vi "tag select data type change.vi"(8 "error in":errorcluster, 9 "Dt Value":i32, 10 "tag select":string, 11 "object ref in":T1) -> (0 "error out":errorcluster, 3 "object ref out":T1)   [LabVIEW 2013, in "tag select module editor node.lvclass"]
uses:
  tag select module editor node.lvclass
  object ref.ctl
  <vilib>/NI/Tag Bus Data Framework/Configuration Editor/Classes/Engine Parent/Engine Parent Editor Node.lvclass
  module/configuration/tag select module configuration.lvclass
  <vilib>/NI/Configuration Framework/serializable configuration/NISE_CEF_serializable configuration.lvclass/NISE_CEF_serializable configuration.ctl
  <vilib>/Utility/LVClass/Get LV Class Name.vi
  <vilib>/NI/Configuration Framework/error generator/NISE_error generator.vi
  <vilib>/NI/Module Execution Interface/Engine Configuration/engine configuration.lvclass
  <vilib>/NI/Configuration Framework/serializable configuration/NISE_CEF_serializable configuration.lvclass
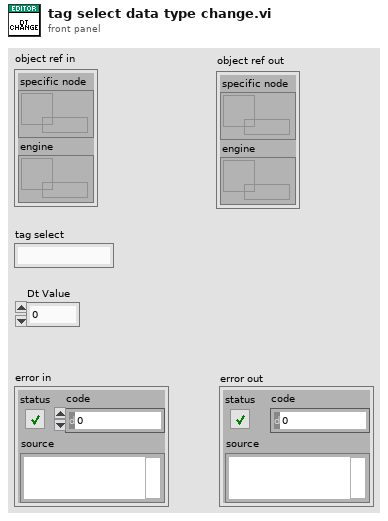
[diagram p1: front panel]
types:
  T1 = typedef "tag select module editor node.lvclass/object ref.ctl" = cluster{"specific node":refnum<data-value>, "engine":refnum<data-value>}
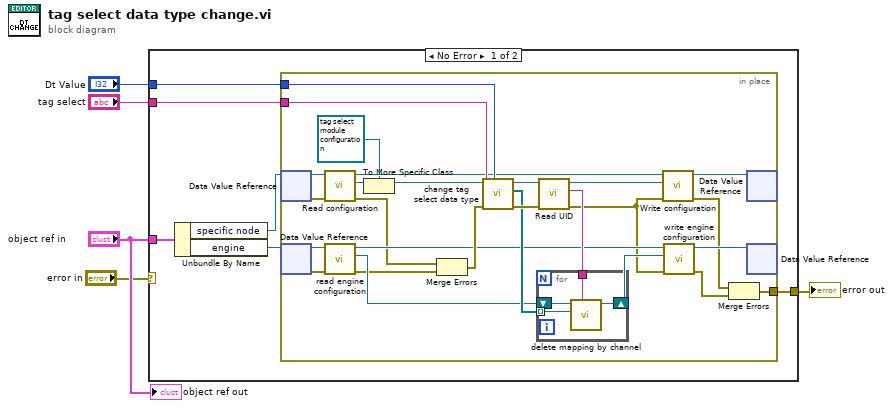
[diagram p0: block diagram]
diagram:
  n1 = case shown="No Error" "error in" {
    selector: "error in" -> [_ w43]
    tunnel: "object ref in" -> [w9 _]
    tunnel: [w8 w43] -> w4
    tunnel: "tag select" -> [w7 _]
    tunnel: "Dt Value" -> [w6 _]
    frame No Error {
      n2 = Unbundle By Name(w9) -> ("specific node"=w10:refnum<data-value>, "engine"=w11:refnum<data-value>)
      n3 = in-place {
        in-place-border: [w19] -> w8
        in-place-border: w7 -> [w36]
        in-place-border: w6 -> [w34]
        n4 = in-place-dvr #1(w10) -> (w12:refnum<class "tag select module editor node.lvclass">, w18:errorcluster)
        n5 = in-place-dvr #2(w11) -> (w37:refnum<class "Engine Parent Editor Node.lvclass">, w38:errorcluster)
        n6 = call-dynamic "Read configuration.vi"("error in"=w18, "tag select module editor node in"=w12) -> ("error out"=w17:errorcluster, "configuration"=w14:refnum<class "NISE_CEF_serializable configuration.lvclass">, "tag select module editor node out"=w23:refnum<class "tag select module editor node.lvclass">)  [unwired: 7 in]
        n7 = call <vilib>:"read engine configuration.vi"("error in"=w38, "Engine Parent Editor Node in"=w37) -> ("error out"=w26:errorcluster, "engine configuration"=w27:refnum<class "engine configuration.lvclass">, "Engine Parent Editor Node out"=w24:refnum<class "Engine Parent Editor Node.lvclass">)  [unwired: 7 in]
        n8 = To More Specific Class(target class=refnum<class "tag select module configuration.lvclass"> refnum ("tag select  module configuration in"), reference=w14) -> (specific class reference=w13:refnum<class "tag select module configuration.lvclass">)  [unwired: 1 in, 1 out]
        n9 = Merge Errors(w17, w26) -> (w32:errorcluster)
        n10 = call "change tag select data type.vi"("data type"=w34, "error in"=w32, "tag select name"=w36, "tag select  module configuration in"=w13) -> ("error out"=w31:errorcluster, "changed channels"=w30:refnum<class "TBM channel.lvclass">[], "tag select module configuration out"=w29:refnum<class "tag select module configuration.lvclass">)  [unwired: 5 in]
        n11 = call <vilib>:"Read UID.vi"("error in"=w31, "configuration in"=w29) -> ("error out"=w16:errorcluster, "instance id"=w28:string, "configuration out"=w22:refnum<class "tag select module configuration.lvclass">)  [unwired: 7 in]
        n12 = for {
          shift-right: [w42] -> w25
          shift-left: w27 -> [w41]
          tunnel: w30 -> [w40] mode=indexing
          tunnel: w28 -> [w39]
          n13 = call <vilib>:"delete mapping by channel.vi"("owner ID"=w39, "channel"=w40, "engine configuration in"=w41) -> ("engine configuration out"=w42:refnum<class "engine configuration.lvclass">)  [unwired: 7 in, 1 out]
        }
        n14 = call-dynamic "Write configuration.vi"("error in"=w16, "configuration"=w22, "tag select module editor node in"=w23) -> ("error out"=w20:errorcluster, "tag select module editor node out"=w33:refnum<class "tag select module editor node.lvclass">)  [unwired: 7 in]
        n15 = call <vilib>:"write engine configuration.vi"("error in"=w16, "engine configuration"=w25, "Engine Parent Editor Node in"=w24) -> ("error out"=w21:errorcluster, "Engine Parent Editor Node out"=w35:refnum<class "Engine Parent Editor Node.lvclass">)  [unwired: 7 in]
        n16 = Merge Errors(w20, w21) -> (w19:errorcluster)
        n17 = in-place-dvr #1(w33) -> ()  [unwired: 2 out]
        n18 = in-place-dvr #2(w35) -> ()  [unwired: 2 out]
      }
    }
    frame Error {
    }
  }
  "error out" <- w4
  "object ref out" <- "object ref in"
